vi "stop.vi"(3 "error in (no error)":errorcluster, 4 "stop":bool, 5 "SoundAO in":refnum<class "SoundAO.lvclass">) -> (0 "error out":errorcluster, 1 "Stopped":bool, 2 "SoundAO out":refnum<class "SoundAO.lvclass">)   [LabVIEW 2009, in "Hardware.lvlib" / "Channels.lvlib" / "SoundAO.lvclass"]
doc: "Abstract Method.\n\nStops the analog output. This vi indicates of the analog output has stopped, and can be used to actively stop the output."
uses:
  SoundAO.lvclass
  SoundAO.lvclass/SoundAO.ctl
  AnalogOutput.lvclass
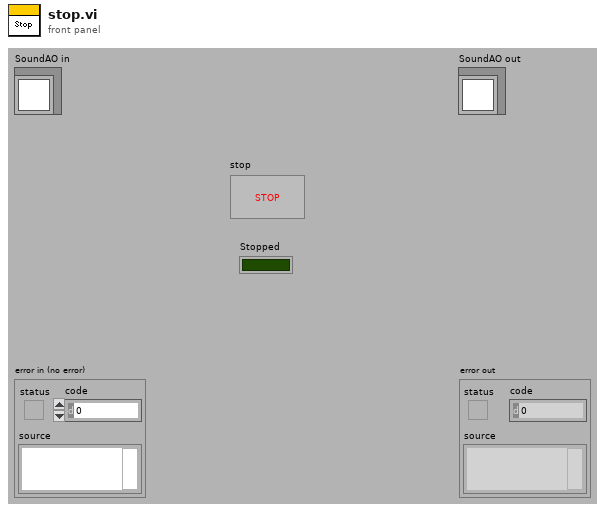
[diagram p1: front panel]
types:
  T1 = typedef "Sound Output Task ID.ctl" = u32
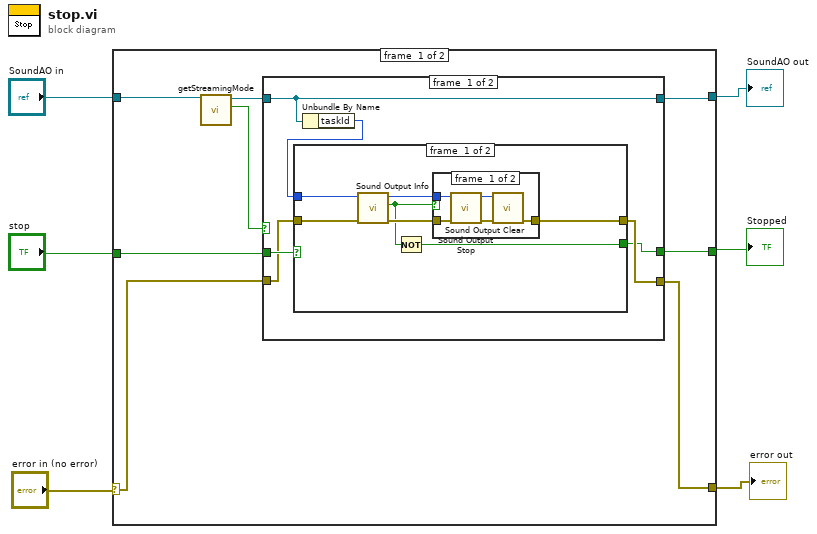
[diagram p0: block diagram]
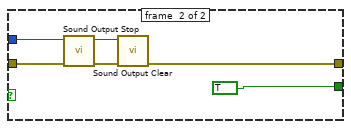
[diagram p3: hidden frame]
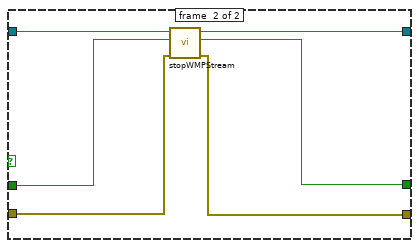
[diagram p4: hidden frame]
diagram:
  n1 = case shown="No Error" "error in (no error)" {
    selector: "error in (no error)" -> [w13 w47]
    tunnel: "SoundAO in" -> [w10 w46]
    tunnel: [w12 w47] -> w4
    tunnel: [w7 w46] -> w3
    tunnel: "stop" -> [w14 _]
    tunnel: [w11 _] -> w1
    frame #0 {
      n2 = call "getStreamingMode.vi"("AnalogOutput.lvclass in"=w10) -> ("streamingMode"=w9:bool, "AnalogOutput.lvclass out"=w8:refnum<class "SoundAO.lvclass">)  [unwired: 8 in, 1 out]
      n3 = case shown="True" w9 {
        tunnel: w14 -> [w20 w40]
        tunnel: w13 -> [w19 w43]
        tunnel: [w18 w42] -> w12
        tunnel: [w17 w41] -> w11
        tunnel: [w16 w44] -> w7
        tunnel: w8 -> [w16 w45]
        frame #0 {
          n4 = Unbundle By Name(w16) -> ("taskId"=w15:i32)
          n5 = case shown="False" w20 {
            tunnel: w15 -> [w26 w37]
            tunnel: w19 -> [w27 w36]
            tunnel: [w25 w35] -> w18
            tunnel: [w24 TRUE] -> w17
            frame #0 {
              n6 = call <vilib>:"Sound Output Info.vi"("error in (no error)"=w27, "task ID"=w26) -> ("error out"=w22:errorcluster, "is playing?"=w21:bool, "task ID out"=w23:T1)  [unwired: 6 in, 1 out]
              n7 = Not(x=w21) -> (.not. x?=w24:bool)
              n8 = case shown="False" w21 {
                tunnel: w23 -> [w29 _]
                tunnel: w22 -> [w28 w33]
                tunnel: [w30 w33] -> w25
                frame #0 {
                  n9 = call <vilib>:"Sound Output Stop.vi"("error in (no error)"=w28, "task ID"=w29) -> ("error out"=w31:errorcluster, "task ID out"=w32:T1)  [unwired: 8 in]
                  n10 = call <vilib>:"Sound Output Clear.vi"("error in (no error)"=w31, "task ID"=w32) -> ("error out"=w30:errorcluster)  [unwired: 9 in]
                }
                frame #1 {
                }
              }
            }
            frame #1 {
              n11 = call <vilib>:"Sound Output Stop.vi"("error in (no error)"=w36, "task ID"=w37) -> ("error out"=w38:errorcluster, "task ID out"=w39:T1)  [unwired: 8 in]
              n12 = call <vilib>:"Sound Output Clear.vi"("error in (no error)"=w38, "task ID"=w39) -> ("error out"=w35:errorcluster)  [unwired: 9 in]
            }
          }
        }
        frame #1 {
          n13 = call "stopWMPStream.vi"("error in (no error)"=w43, "stop"=w40, "SoundAO in"=w45) -> ("error out"=w42:errorcluster, "Stopped"=w41:bool, "SoundAO out"=w44:refnum<class "SoundAO.lvclass">)  [unwired: 6 in]
        }
      }
    }
    frame #1 {
    }
  }
  "error out" <- w4
  "SoundAO out" <- w3
  "Stopped" <- w1
